vi "Find Nodes Attribute.vi"(8 "error in (no error)":errorcluster, 10 "XPath":T1, 11 "Node in":refnum<k20>) -> (0 "error out":errorcluster, 2 "Attribute":string[](array[string]), 3 "Node out":refnum<k20>)   [LabVIEW 2020, in "VI Properties Editor.lvlib"]
doc: "Finds attributes in <B>Node in</B>, given <B>XPath</B>."
uses:
  VI Properties Editor.lvlib
  <resource>/objmgr/DOMUserDefRef.rc
  <vilib>/xml/NI_XML.lvlib
  CTLs/XPath Get Attribute.ctl
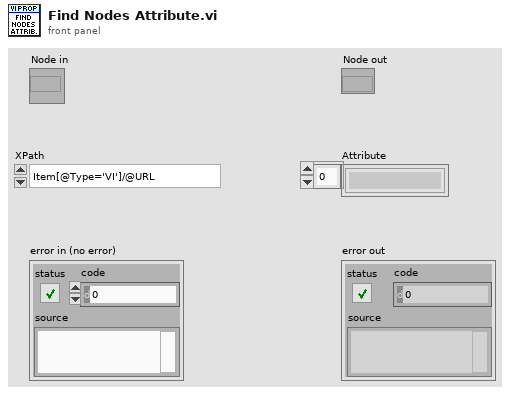
[diagram p1: front panel]
types:
  T1 = typedef "VI Properties Editor.lvlib/XPath Get Attribute.ctl" = enum16{"Item[@Type='VI']/@URL", "Item[@Type='LVClass']/@URL", "Item[@Type='Library']/@URL", "Item[@Type='Folder' and not (@URL)]/@Name", "@Name"}
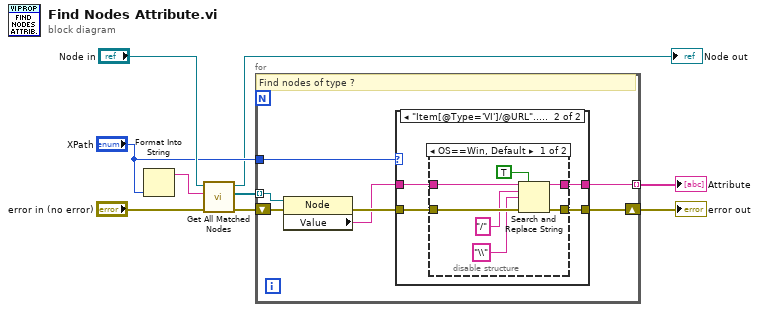
[diagram p0: block diagram]
diagram:
  n1 = Format Into String("XPath") -> (resulting string=w4:string)  [unwired: 3 in, 1 out]
  n2 = call <vilib>:"Get All Matched Nodes.vi"("error in (no error)"="error in (no error)", "XPath expression"=w4, "node in"="Node in") -> ("error out"=w9:errorcluster, "node result array"=w6:refnum<k20>[], "node out"=→"Node out":refnum<k20>)  [unwired: 6 in]
  n3 = for {
    tunnel: w6 -> [w13] mode=indexing
    tunnel: [w12] -> w5 mode=indexing
    shift-right: [w15] -> w7
    shift-left: w9 -> [w16]
    tunnel: "XPath" -> [w10]
    # "Find nodes of type ?"
    n4 = property on="Property Node" class="Node"(reference=w13, error in=w16) -> (error out=w14:errorcluster, "Value"=w11:string)  [unwired: 1 out]
    n5 = case shown="\"Item[@Type='VI']/@URL\"..\"Item[@Type='Library']/@URL\"" w10 {
      tunnel: [w17 w20] -> w12
      tunnel: [w18 w22] -> w15
      tunnel: w14 -> [w18 w21]
      tunnel: w11 -> [w17 w19]
      frame "@Name", Default {
      }
      frame "Item[@Type='VI']/@URL".."Item[@Type='Library']/@URL" {
        n6 = disable-structure "Conditional Disable Structure" shown="OS==Win, Default" {
          disable-tunnel: [w27 w30] -> w20
          disable-tunnel: w19 -> [w26 w30]
          disable-tunnel: w21 -> [w29 w31]
          disable-tunnel: [w28 w31] -> w22
          frame condition #0 (active) {
            n7 = Search and Replace String(replace all?=TRUE ("replace all? (F)"), input string=w26, search string="/", replace string="\\" ("replace string (\"\")"), error in=w29) -> (result string=w27:string, error out=w28:errorcluster)  [unwired: 3 in, 2 out]
          }
          frame condition #1 {
          }
        }
      }
    }
  }
  "Attribute" <- w5
  "error out" <- w7
